vi "logging_session_set_parameter.vi"(7 "Logging Parameter":T1, 8 "error in":errorcluster, 9 "String parameter (\"\")":string, 10 "I32 parameter (0)":i32, 11 "VISA resource name":refnum<visa-resource-name>) -> (0 "error out":errorcluster, 3 "VISA resource name out":refnum<visa-resource-name>)   [LabVIEW 2014, in "rszvl_rsidr_core.lvlib"]
uses:
  rszvl_rsidr_core.lvlib
  type_Logging_Parameter.ctl
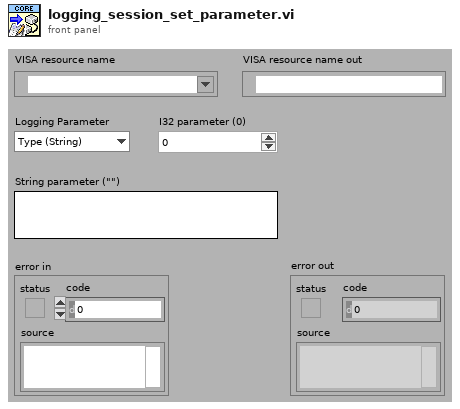
[diagram p1: front panel]
types:
  T1 = typedef "rszvl_rsidr_core.lvlib/type_Logging_Parameter.ctl" = enum16{"Type (String)", "SessionAlias(String)", "FormatString (String)", "UDPconectionID (I32)", "UDPlocalPort (I32)", "UDPremotePort (I32)", "UDPremoteHost (String)", "FILEmode (I32)", "FILEpath (String)", "FILEopenID (I32)"}
  T2 = typedef "rszvl_rsidr_core.lvlib/type_Session_Data.ctl" = cluster{"Instr type":string, "Instr type for err. msg.":string, "Installed Options":string[], "OPC Timeout":i32, "Query Instrument Status":bool, "Check Range":bool, "Check Options":bool, "Add LF to Write":bool, "Simulate":bool, "Logging":bool, "Logging params":variant, "Interface Type":enum16{"Unknown", "GPIB", "VXI", "GPIB_VXI", "ASRL", "PXI", "TCPIP", "USB", "SOCKET"}, "Fast Sweep":i32, "AdditionalFlags":i32, "WaitBeforeWrite":i32, "WaitBeforeRead":i32, "BinDataChunkSize":i64}
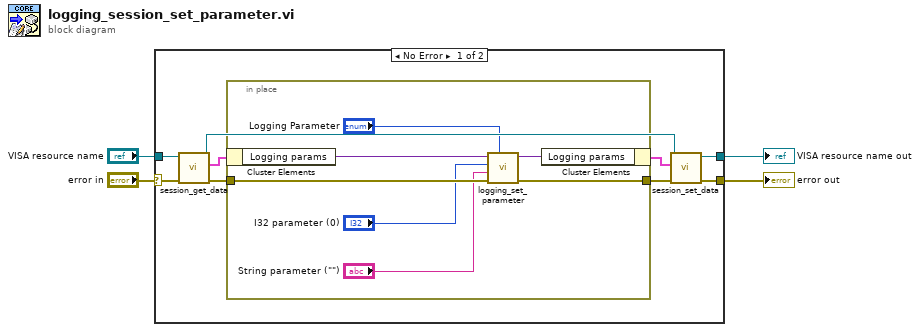
[diagram p0: block diagram]
diagram:
  n1 = case shown="No Error" "error in" {
    selector: "error in" -> [w13 w22]
    tunnel: "VISA resource name" -> [w12 w21]
    tunnel: [w9 w22] -> w3
    tunnel: [w8 w21] -> w1
    frame No Error {
      n2 = call "session_get_data.vi"("error in"=w13, "VISA resource name"=w12) -> ("error out"=w11:errorcluster, "Session User Data out"=w5:T2, "VISA resource name out"=w6:refnum<visa-resource-name>)  [unwired: 7 in]
      n3 = in-place "In Place Element Structure" {
        in-place-border: w11 -> [w20]
        in-place-border: [w19] -> w10
        n4 = in-place-cluster #1 ("Unbundle / Bundle Elements")(w5) -> ("Logging params"=w16:variant)
        n5 = call "logging_set_parameter.vi"("Logging Parameter"="Logging Parameter", "error in"=w20, "String parameter (\"\")"="String parameter (\"\")", "I32 parameter (0)"="I32 parameter (0)", "Logging params in"=w16) -> ("error out"=w19:errorcluster, "Logging params out"=w15:variant)  [unwired: 5 in]
        n6 = in-place-cluster #1 ("Unbundle / Bundle Elements")("Logging params"=w15) -> (w7:T2)
      }
      n7 = call "session_set_data.vi"("error in"=w10, "Session User Data in"=w7, "VISA resource name"=w6) -> ("error out"=w9:errorcluster, "VISA resource name out"=w8:refnum<visa-resource-name>)  [unwired: 7 in]
    }
    frame Error {
    }
  }
  "VISA resource name out" <- w1
  "error out" <- w3
